vi "ImagePath(SubVI).vi"(11 "Name":string) -> (3 "ImagePath":path)   [LabVIEW 2013]
uses:
  <vilib>/Utility/sysdir.llb/System Directory Type.ctl
  Dropbox/Programs/FYP_LabviewGlobal(SubVI).vi
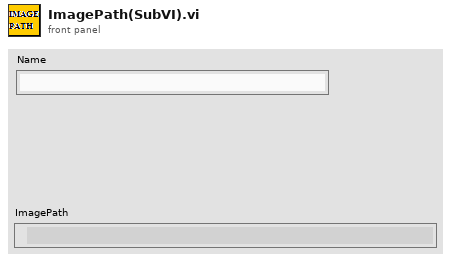
[diagram p1: front panel]
types:
  T1 = typedef "System Directory Type.ctl" = i32
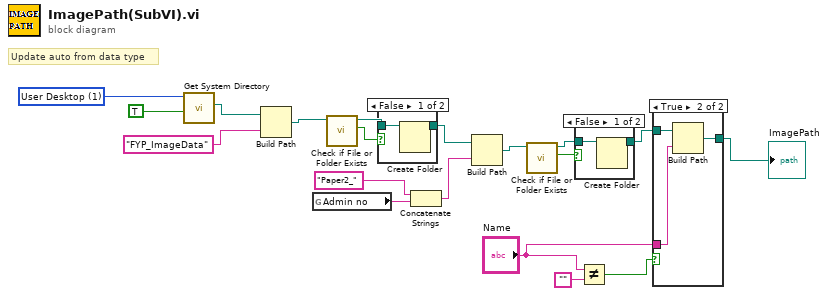
[diagram p0: block diagram]
diagram:
  w19 = T1 1 items=["User Home"=0, "User Desktop"=1, "User Documents"=2, "User Application Data"=3, "User Preferences"=4, "User Temporary"=5, "Public Documents"=6, "Public Application Data"=7, "Public Preferences"=8, "Public Cache"=13, "System Core Libraries"=9, "System Installed Libraries"=10, "Application Files"=11, "Boot Volume Root"=12] ("system directory type")
  # "Update auto from data type"
  n1 = call <vilib>:"Get System Directory.vi"("create directory if not found? (F)"=TRUE, "system directory type"=w19) -> ("system directory"=w17:path)  [unwired: 9 in]
  n2 = Build Path(base path=w17, name or relative path="FYP_ImageData") -> (appended path=w15:path)
  n3 = global read "FYP_LabviewGlobal(SubVI).vi" "Admin no"() -> (w4:string)
  n4 = call <vilib>:"Check if File or Folder Exists.vi"("path"=w15) -> ("file or folder exists?"=w13:bool, "dup path"=w14:path)  [unwired: 8 in, 1 out]
  n5 = case shown="False" w13 {
    tunnel: w14 -> [w21 w22]
    tunnel: [w20 w22] -> w8
    frame False {
      n6 = Create Folder(path (use dialog)=w21) -> (created path=w20:path)  [unwired: 2 in, 2 out]
    }
    frame True {
    }
  }
  n7 = Concatenate Strings("Paper2_", w4) -> (w2:string)
  n8 = Build Path(base path=w8, name or relative path=w2) -> (appended path=w9:path)
  n9 = call <vilib>:"Check if File or Folder Exists.vi"("path"=w9) -> ("file or folder exists?"=w6:bool, "dup path"=w7:path)  [unwired: 8 in, 1 out]
  n10 = case shown="False" w6 {
    tunnel: w7 -> [w24 w25]
    tunnel: [w23 w25] -> w5
    frame False {
      n11 = Create Folder(path (use dialog)=w24) -> (created path=w23:path)  [unwired: 2 in, 2 out]
    }
    frame True {
    }
  }
  n12 = Not Equal?(x="Name", y="") -> (x != y?=w10:bool)
  n13 = case shown="True" w10 {
    tunnel: [w26 w29] -> w1
    tunnel: w5 -> [w26 w28]
    tunnel: "Name" -> [_ w27]
    frame False {
    }
    frame True {
      n14 = Build Path(base path=w28, name or relative path=w27) -> (appended path=w29:path)
    }
  }
  "ImagePath" <- w1
